vi "log_main.vi"(7 "FGV_mods":T1, 8 "Error In":errorcluster, 11 "DataIn":variant) -> (0 "Error Out":errorcluster)   [LabVIEW 2017]
uses:
  log_mods.ctl
  log_data.ctl
  log_status.ctl
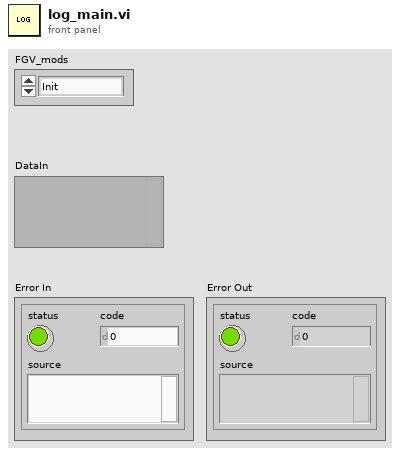
[diagram p1: front panel]
types:
  T1 = typedef "log_mods.ctl" = enum16{"Init", "SetStatus", "RMSacel", "HitData", "Clear", "PeakForce", "WriteToLog", "End"}
  T2 = typedef "log_data.ctl" = cluster{"log_status":T3, "RMS_acel":dbl[], "LogRef":refnum<vi>, "log_file":refnum<file>, "hammerPeak":dbl, "peakFreqs":dbl[], "hits":i32, "hit":bool}
  T3 = typedef "log_status.ctl" = enum16{"Init", "Ready", "Running", "Error", "End"}
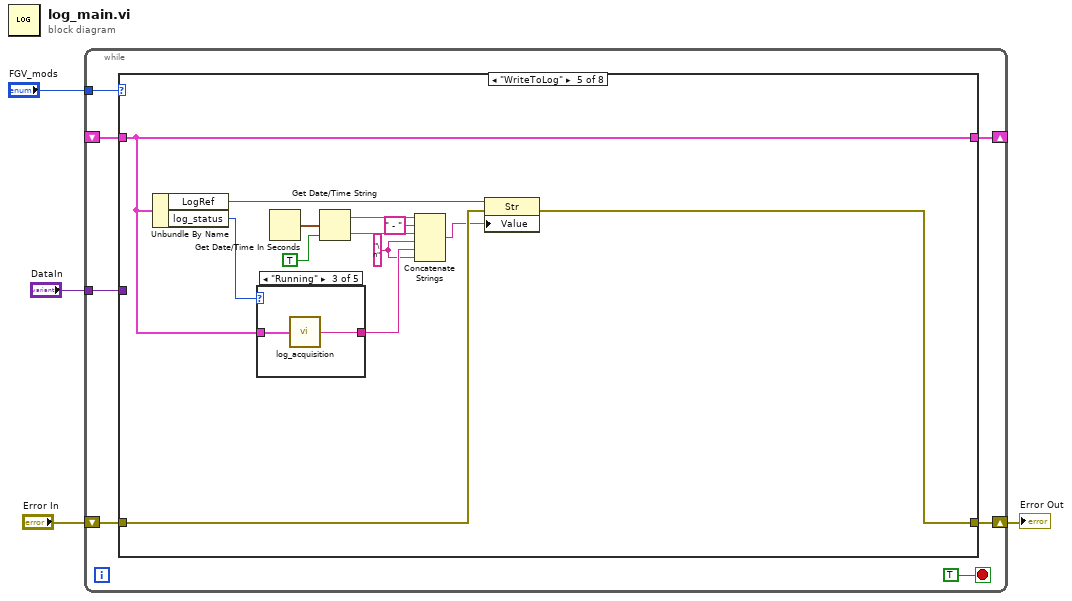
[diagram p0: block diagram]
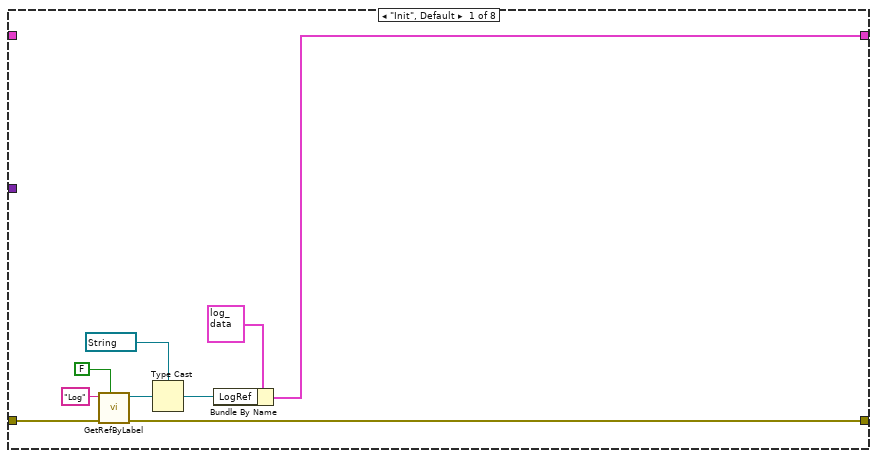
[diagram p2: hidden frame]
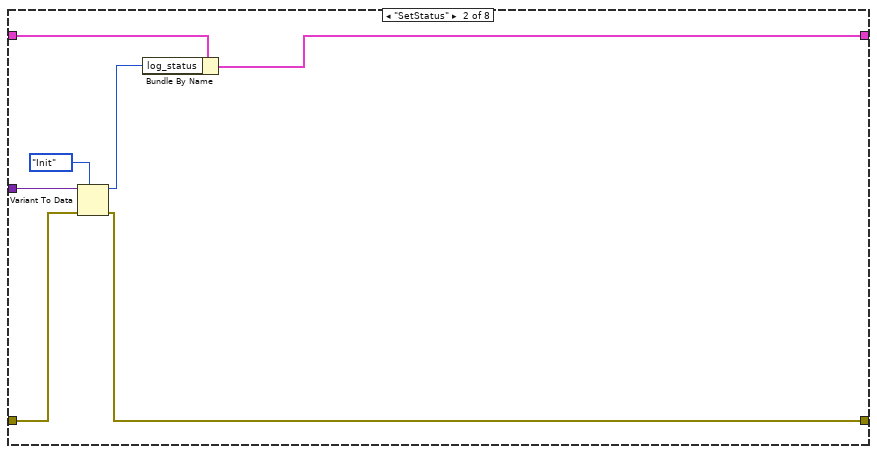
[diagram p3: hidden frame]
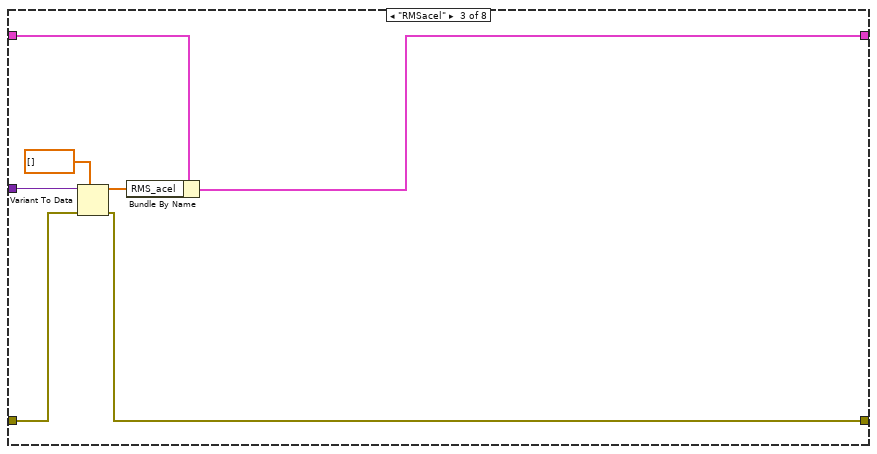
[diagram p4: hidden frame]
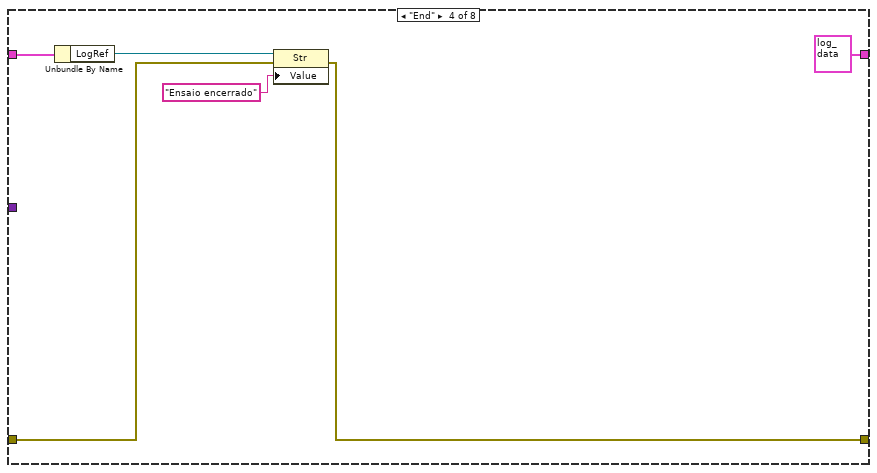
[diagram p5: hidden frame]
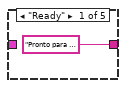
[diagram p6: hidden frame]
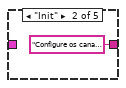
[diagram p7: hidden frame]
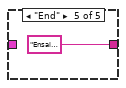
[diagram p9: hidden frame]
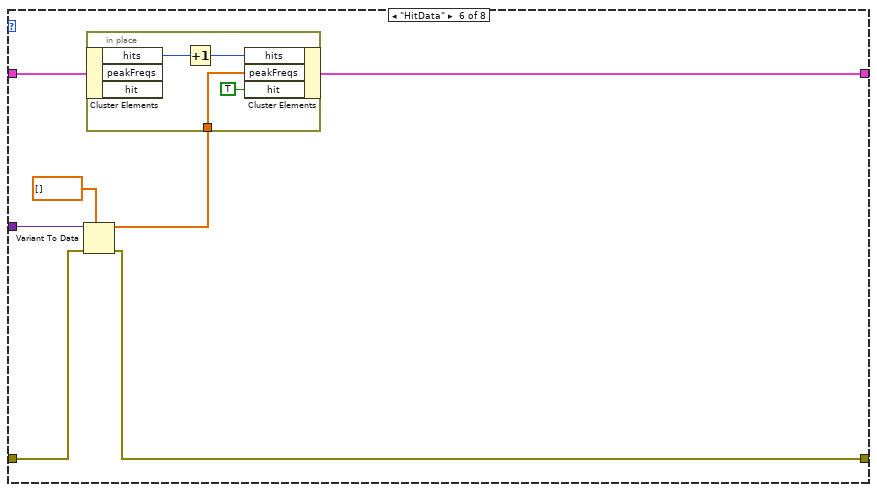
[diagram p10: hidden frame]
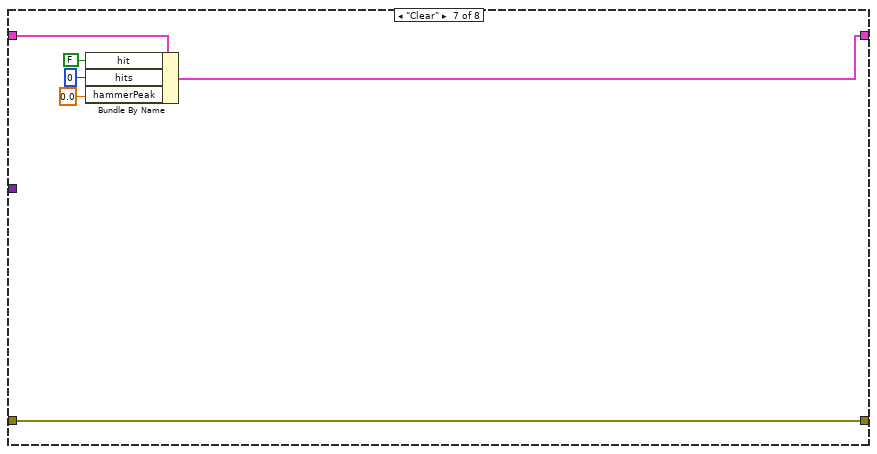
[diagram p11: hidden frame]
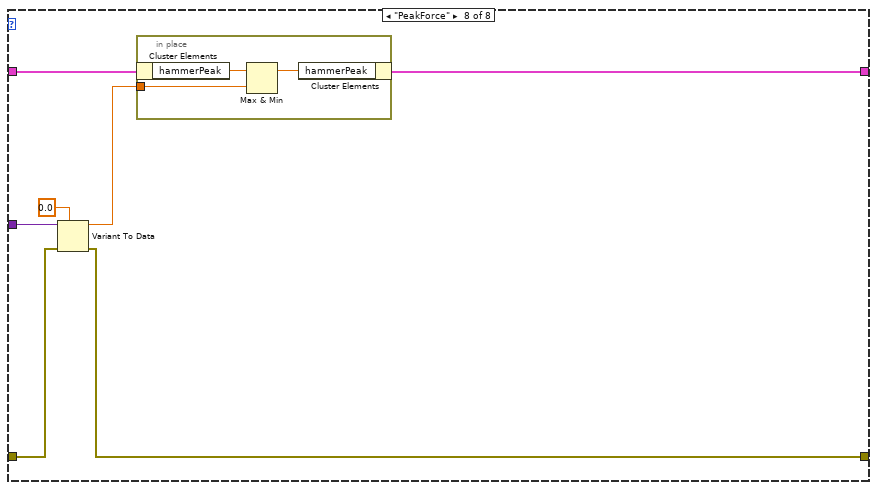
[diagram p12: hidden frame]
diagram:
  n1 = while {
    tunnel: "DataIn" -> [w10]
    tunnel: "FGV_mods" -> [w9]
    shift-right: [w8] -> _
    shift-left: _ -> [w7]
    shift-right: [w5] -> w1
    shift-left: "Error In" -> [w6]
    stop <- TRUE stop-if-true
    n2 = case shown="\"WriteToLog\"" w9 {
      tunnel: w10 -> [_ w25 w32 _ _ w64 _ w82]
      tunnel: [w13 w26 w33 T2 {"log_status"=enum."Init", "RMS_acel"=[], "LogRef"=refnum, "log_file"=refnum, "hammerPeak"=0.0, "peakFreqs"=[], "hits"=0, "hit"=FALSE} ("log_data") w52 w59 w71 w77] -> w8
      tunnel: w7 -> [_ w27 w34 w39 w52 w65 w75 w79]
      tunnel: w6 -> [w18 w24 w31 w36 w50 w63 w70 w80]
      tunnel: [w12 w21 w30 w35 w41 w62 w70 w76] -> w5
      frame "Init", Default {
        n3 = call "GetRefByLabel.vi"("InsideTab"=FALSE, "error in"=w18, "Label"="Log") -> ("error out"=w12:errorcluster, "Ctl Refnum"=w17:refnum<vi>)  [unwired: 6 in, 1 out]
        n4 = Type Cast(type=refnum<vi> refnum ("Log"), x=w17) -> (*(type *) &x=w14:refnum<vi>)
        n5 = Bundle By Name(cluster=T2 {"log_status"=enum."Init", "RMS_acel"=[], "LogRef"=refnum, "log_file"=refnum, "hammerPeak"=0.0, "peakFreqs"=[], "hits"=0, "hit"=FALSE} ("log_data"), "LogRef"=w14) -> (w13:T2)
      }
      frame "SetStatus" {
        n6 = Variant To Data(error in=w24, type=log_status."Init" ("log_status"), Variant=w25) -> (data=w22:T3, error out=w21:errorcluster)
        n7 = Bundle By Name(cluster=w27, "log_status"=w22) -> (w26:T2)
      }
      frame "RMSacel" {
        n8 = Variant To Data(error in=w31, type=dbl[] [] ("SG_data"), Variant=w32) -> (data=w28:dbl[], error out=w30:errorcluster)
        n9 = Bundle By Name(cluster=w34, "RMS_acel"=w28) -> (w33:T2)
      }
      frame "End" {
        n10 = Unbundle By Name(w39) -> ("LogRef"=w38:refnum<vi>)
        n11 = property class="Str"(reference=w38, error in=w36, "Value"="Ensaio encerrado") -> (error out=w35:errorcluster)  [unwired: 1 out]
      }
      frame "WriteToLog" {
        w42 = "\n" ("string")
        n12 = Unbundle By Name(w52) -> ("LogRef"=w51:refnum<vi>, "log_status"=w53:T3)
        n13 = case shown="\"Running\"" w53 {
          tunnel: w52 -> [_ _ w57 _ _]
          tunnel: ["Pronto para o início do ensaio" ("Value") "Configure os canais antes do início do ensaio" ("Value") w56 _ "Ensaio encerrado" ("Value")] -> w45
          frame "Ready" {
          }
          frame "Init" {
          }
          frame "Running" {
            n14 = call "log_acquisition.vi"("log_data"=w57) -> ("Log"=w56:string)
          }
          frame "Error" {
          }
          frame "End" {
          }
        }
        n15 = Get Date/Time In Seconds() -> (seconds since 1Jan1904=w49:timestamp)
        n16 = Get Date/Time String(seconds (now)=w49, want seconds? (F)=TRUE) -> (date string=w48:string, time string=w47:string)  [unwired: 1 in]
        n17 = Concatenate Strings(w48, " - " ("string"), w47, w42, w45, w42) -> (w43:string)
        n18 = property class="Str"(reference=w51, error in=w50, "Value"=w43) -> (error out=w41:errorcluster)  [unwired: 1 out]
      }
      frame "HitData" {
        n19 = Variant To Data(error in=w63, type=dbl[] [], Variant=w64) -> (data=w60:dbl[], error out=w62:errorcluster)
        n20 = in-place {
          in-place-border: w60 -> [w67]
          n21 = in-place-cluster #1(w65) -> ("hits"=w69:i32)  [unwired: 2 out]
          n22 = Increment(x=w69) -> (x+1=w68:i32)
          n23 = in-place-cluster #1("hits"=w68, "peakFreqs"=w67, "hit"=TRUE) -> (w59:T2)
        }
      }
      frame "Clear" {
        n24 = Bundle By Name(cluster=w75, "hit"=FALSE, "hits"=0, "hammerPeak"=0.0) -> (w71:T2)
      }
      frame "PeakForce" {
        n25 = Variant To Data(error in=w80, type=0.0, Variant=w82) -> (data=w78:dbl, error out=w76:errorcluster)
        n26 = in-place {
          in-place-border: w78 -> [w84]
          n27 = in-place-cluster #2(w79) -> ("hammerPeak"=w85:dbl)
          n28 = Max & Min(x=w85, y=w84) -> (max(x,y)=w83:dbl)  [unwired: 1 out]
          n29 = in-place-cluster #2("hammerPeak"=w83) -> (w77:T2)
        }
      }
    }
  }
  "Error Out" <- w1
